vi "Top Level FPGA_noLED.vi"() -> ()   [LabVIEW 2012]
uses:
  <vilib>/Platform/TimedLoop/XDataNode/XDataNode.xnode
  <vilib>/Platform/TimedLoop/XDataNode/nitl_modes.ctl
  <vilib>/Platform/TimedLoop/XDataNode/XDNodeRunTimeDep.lvlib
  <vilib>/Platform/TimedLoop/XDataNode/wakeup.ctl
  <vilib>/Platform/TimedLoop/XDataNode/timing_clust.ctl
  <vilib>/rvi/DataTransferAndStorage/Container/Common/niFpgaContainerMetaDataKey.ctl
  <vilib>/rvi/FIFO/Fifo_Types/niFpgaFifoControlLogicControl.ctl
  <vilib>/rvi/Memory/Memory_Types/niFpgaMemoryInterfaceConfiguration.ctl
  <vilib>/rvi/DataTransferAndStorage/Container/Common/niFpgaContainerInitializationParameters.ctl
  <vilib>/rvi/DataTransferAndStorage/Container/Common/niFpgaTransferTypeControl.ctl
  <vilib>/rvi/DataTransferAndStorage/Container/Common/niFpgaContainerArbitrationOptionsControl.ctl
  <vilib>/rvi/DataTransferAndStorage/Container/Common/niFpgaContainerImplementationControl.ctl
  <vilib>/rvi/DataTransferAndStorage/Container/Common/niFpgaDataTypeControl.ctl
  <vilib>/rvi/DataTransferAndStorage/Container/Common/niFpgaContainerState.ctl
  <vilib>/rvi/DataTransferAndStorage/Container/Common/niFpgaContainerSetEmuInfo.vi
  <vilib>/rvi/eio/common/nirviEmuReportErrorAndStop.vi
  <vilib>/rvi/DataTransferAndStorage/Container/Common/niFpgaContainerGetUniqueNameForEmu.vi
  <vilib>/rvi/LocalResourceManager/LocalResourceManager.xnode
  <vilib>/rvi/DataTransferAndStorage/Container/XNode/niFpgaContainer.xnode
  <vilib>/rvi/Memory/Memory_Emulation/nirvimemoryEmulation.vi
  <vilib>/rvi/FIFO/Fifo_Resource/nirvififoEmulationRead.vi
  <vilib>/rvi/DataTransferAndStorage/Register/Emulation/niFpgaRegisterEmulation.vi
  <vilib>/eio/EIONode/EIONode.xnode
  <vilib>/rvi/eio/common/nirviEmuTemplateMethod_errors.vi
  <vilib>/rvi/FIFO/Fifo_Resource/nirvififoEmulationClear.vi
  <vilib>/rvi/FIFO/Fifo_Resource/nirvififoEmulationWrite.vi
panel:
  out "Timestamp":u64
  in  "Stop FPGA and exit":bool
  out "Exited cleanly?":bool
  out "DMA FIFO Timed Out?":bool
  in  "location":i16(ring) items=["Purdue", "NIKHEF", "Zurich", "???"]
  in  "show_trigger_position_for_debugging":bool
  in  "channel 7 on/off":bool
  in  "channel 6 on/off":bool
  in  "channel 5 on/off":bool
  in  "channel 4 on/off":bool
  in  "channel 3 on/off":bool
  in  "channel 1 on/off":bool
  in  "channel 2 on/off":bool
  in  "channel 0 on/off":bool
  in  "initial value":u64
  in  "circular buffer length":u32=1000
  in  "# of pretrigger":u32=20
  out "IO Module\\Pll Unlocked":bool
  out "IO Module\\ADC Error B":bool
  out "IO Module\\ADC Error A":bool
  out "Init Done":bool
  in  "Simulate":bool
  in  "Trigger 4":i16=4000
  in  "Trigger 5":i16=4000
  in  "Trigger 6":i16=4000
  in  "Trigger 7":i16=4000
  in  "Trigger 2":i16=4000
  in  "Trigger 3":i16=4000
  in  "Trigger 1":i16=4000
  in  "Record Size only data":u32=95
  in  "Trigger 0":i16=4000
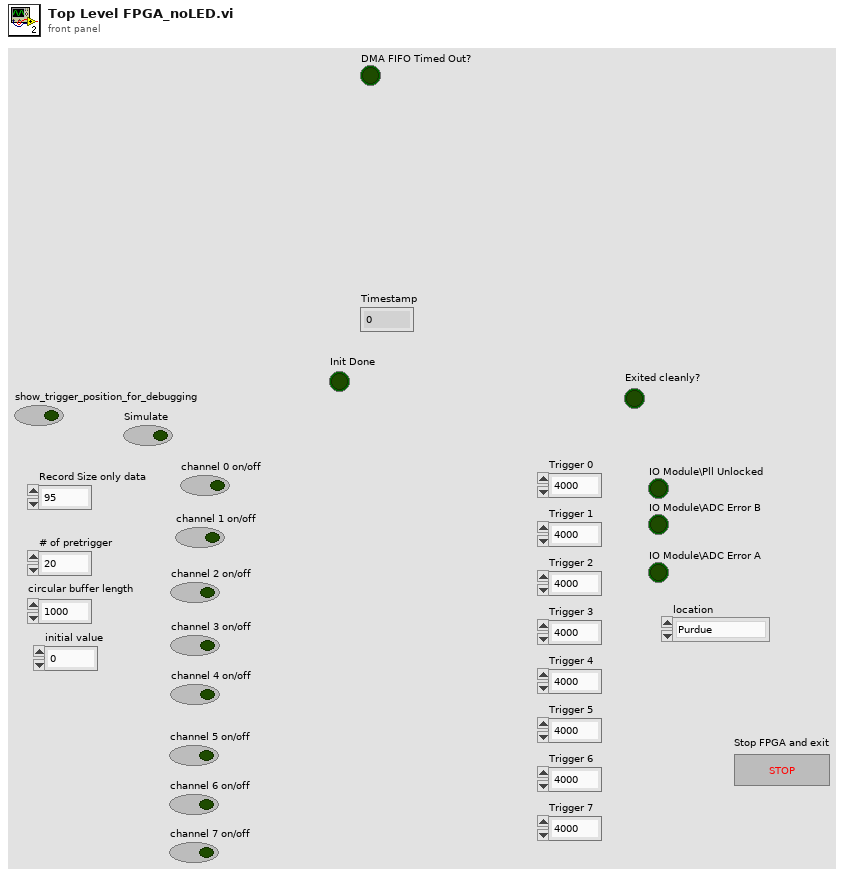
[diagram p1: front panel]
types:
  T1 = typedef "XDNodeRunTimeDep.lvlib/timing_clust.ctl" = cluster{"Expected End [f-1]":u64, "Actual End [f-1]":u64, "Finished Late? [f-1]":bool, "Expected End [i-1]":u64, "Actual End [i-1]":u64, "Finished Late? [i-1]":bool, "Expected Start [i]":u64, "Actual Start [i]":u64, "Expected Start [f]":u64, "Actual Start [f]":u64, "Source Name":string, "Structure Name":string, "Period":i64, "Deadline":i64, "Offset":i64, "Start":i64, "Priority":i32, "Timeout":i32, "Mode":T2, "Wakeup Reason":T3, "Error":errorcluster, "Source Type":string, "Secondary Source Type":string, "Global End Time":u64, "Global Start Time":u64, "Frame Duration":u64, "Iteration Duration":u64, "Assigned CPU":i32, "I/O Scan Engine Mode":u32}
  T2 = typedef "XDNodeRunTimeDep.lvlib/nitl_modes.ctl" = enum32{"No Change", "Process missed periods, maintain original phase", "Discard missed periods, maintain original phase", "Process missed periods, ignore original phase", "Discard missed periods, ignore original phase"}
  T3 = typedef "XDNodeRunTimeDep.lvlib/wakeup.ctl" = enum32{"Normal", "Aborted", "Asynchronous wakeup", "Timing source error", "Timed loop error", "Timeout"}
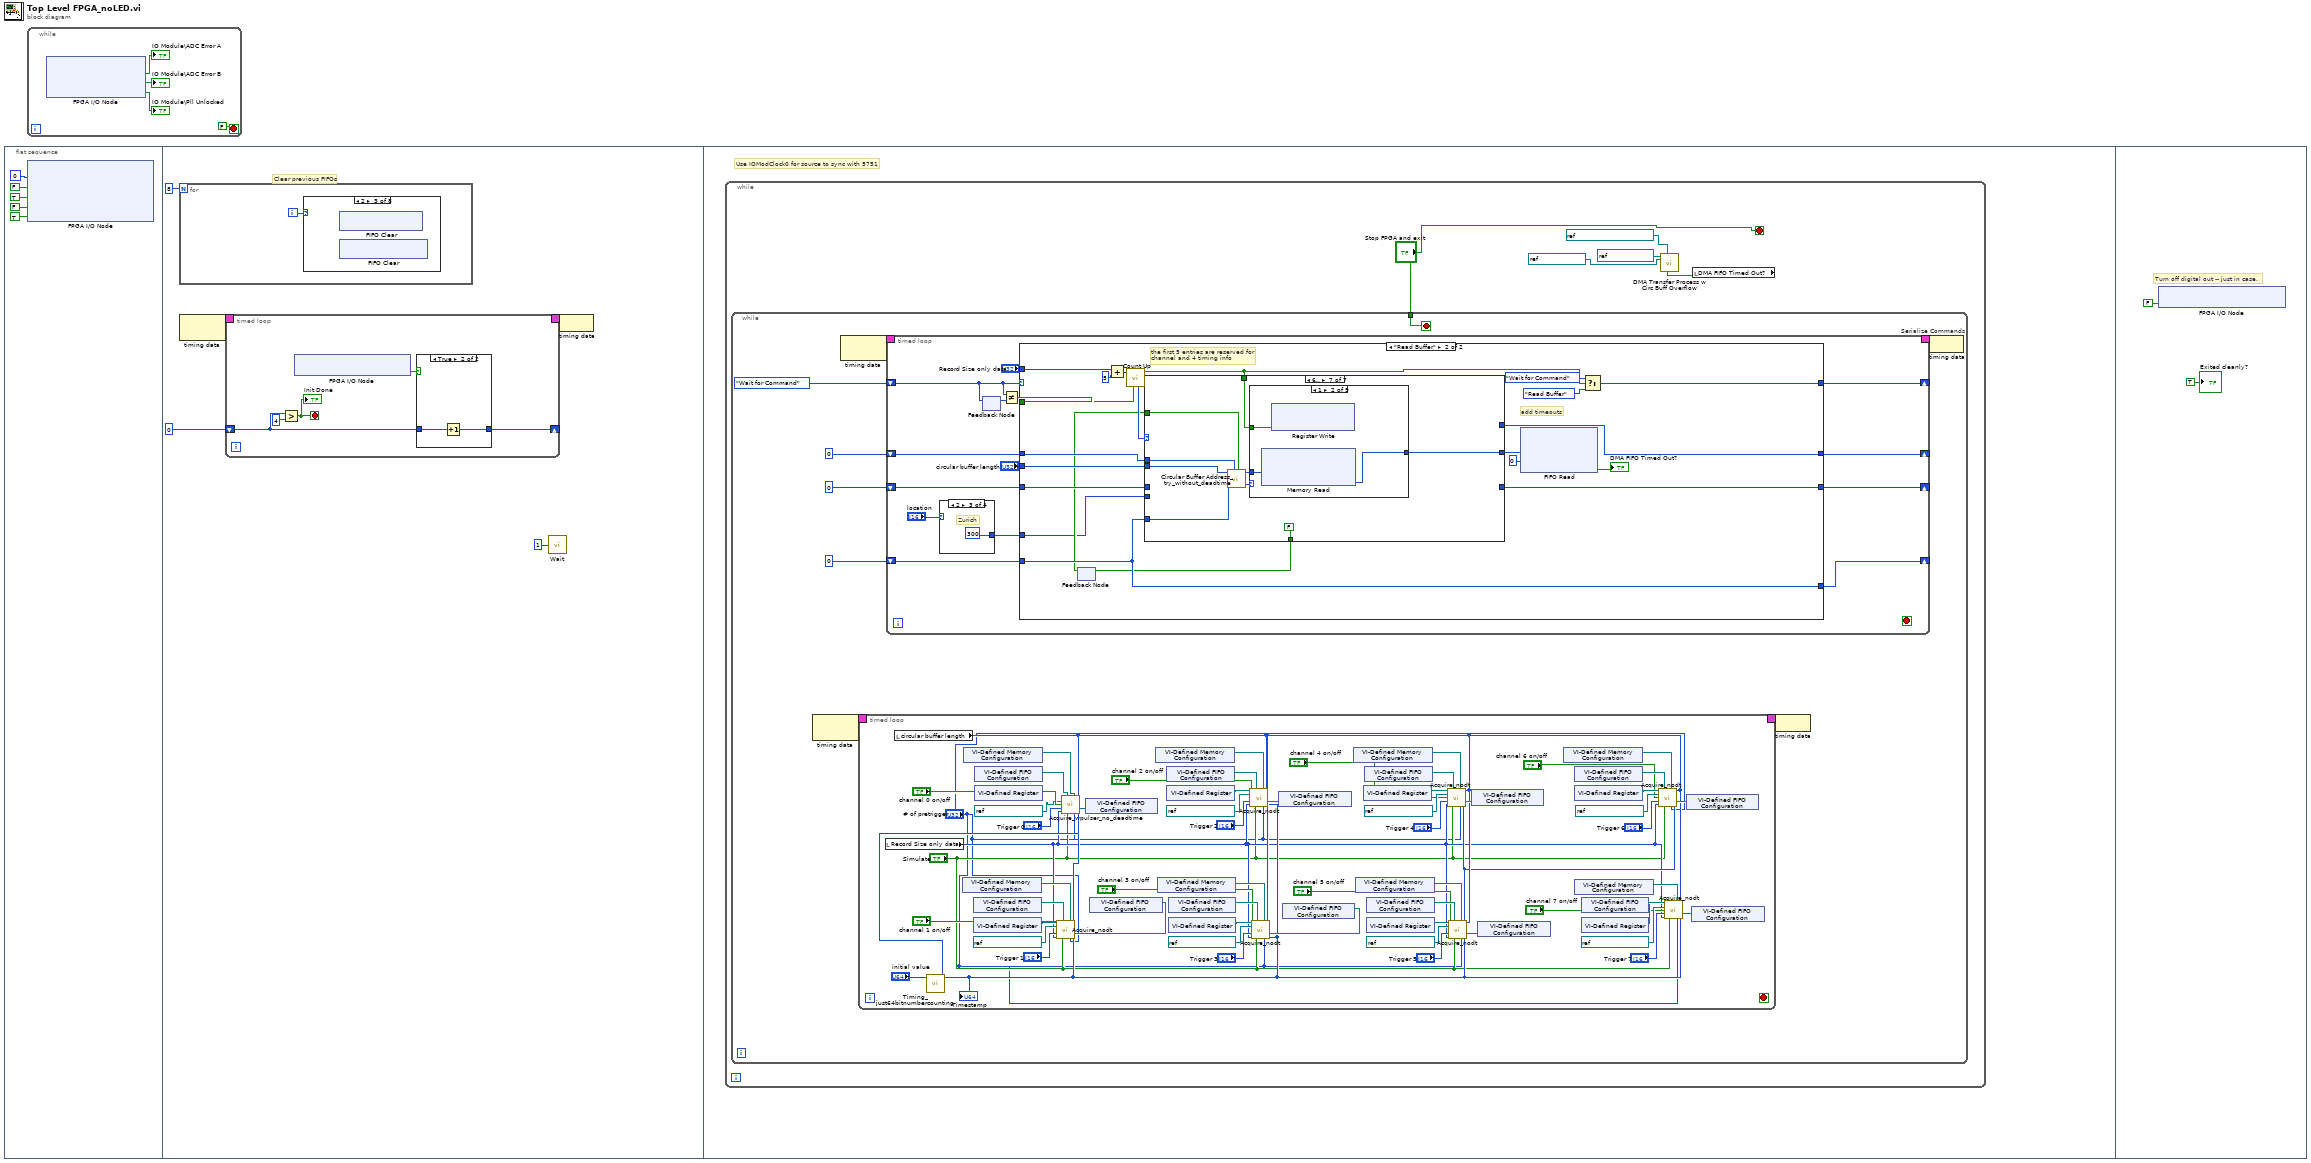
[diagram p0: block diagram]
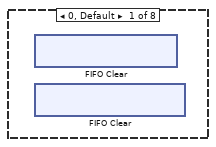
[diagram p2: hidden frame]
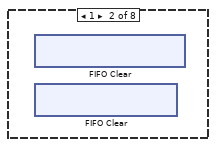
[diagram p3: hidden frame]
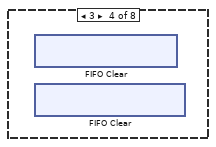
[diagram p4: hidden frame]
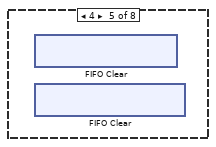
[diagram p5: hidden frame]
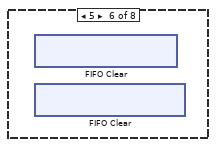
[diagram p6: hidden frame]
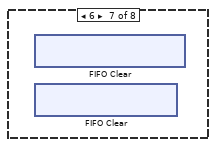
[diagram p7: hidden frame]
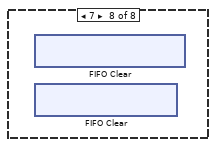
[diagram p8: hidden frame]
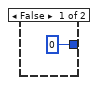
[diagram p9: hidden frame]
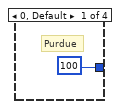
[diagram p10: hidden frame]
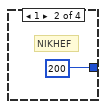
[diagram p11: hidden frame]
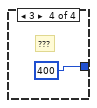
[diagram p12: hidden frame]
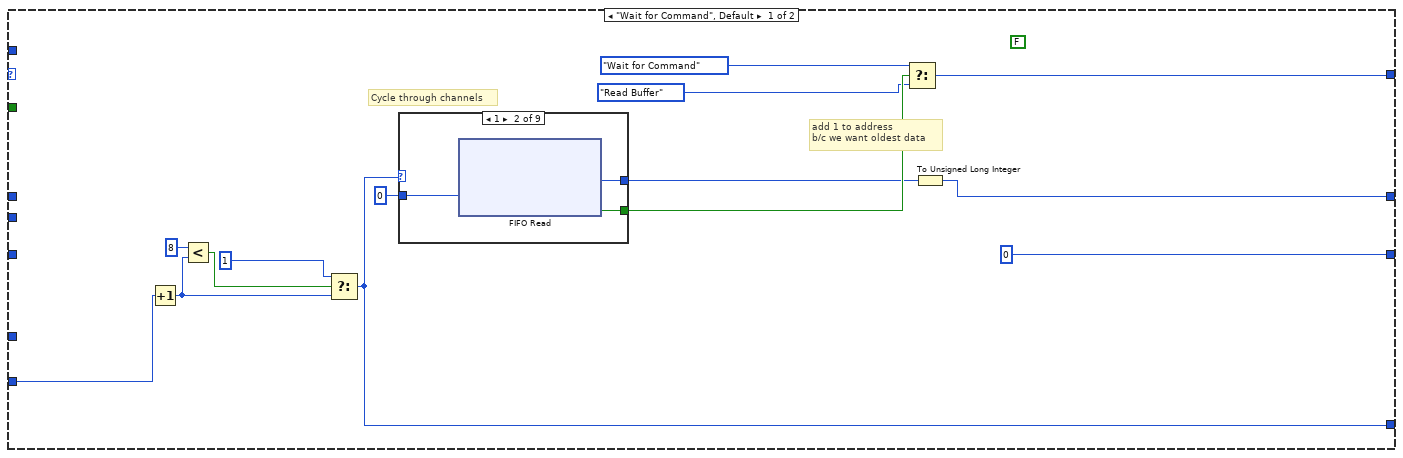
[diagram p13: hidden frame]
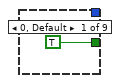
[diagram p14: hidden frame]
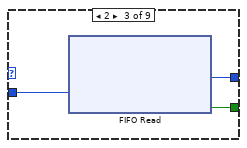
[diagram p15: hidden frame]
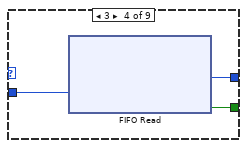
[diagram p16: hidden frame]
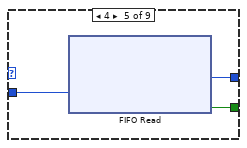
[diagram p17: hidden frame]
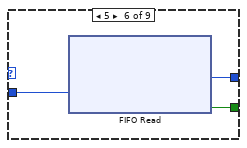
[diagram p18: hidden frame]
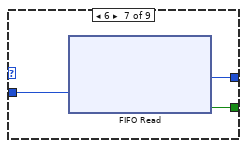
[diagram p19: hidden frame]
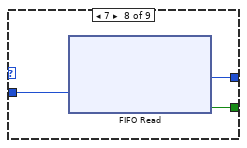
[diagram p20: hidden frame]
diagram:
  n1 = flat-sequence {
    frame #0 {
      n2 = xnode "FPGA I/O Node"("IO Module\\Sample Clock Select"=u8 0 ("IO Module\\Sample Clock Select"), "IO Module\\Force Initialization"=FALSE ("IO Module\\Force Initialization"), "IO Module\\Force Initialization"=TRUE ("IO Module\\Force Initialization"), "IO Module\\Force Initialization"=FALSE ("IO Module\\Force Initialization"), "IO Module\\Digital Output Enable"=TRUE ("IO Module\\Digital Output Enable")) -> ()  [unwired: 5 in, 5 out]
    }
    frame #1 {
      # "Clear previous FIFOs"
      n3 = for {
        N: 8 -> [_]
        i -> [w11]
        n4 = case shown="2" w11 {
          frame 0, Default {
            n5 = xnode ("FIFO Clear")() -> ()  [unwired: 1 in, 1 out]
            n6 = xnode ("FIFO Clear")() -> ()  [unwired: 1 in, 1 out]
          }
          frame 1 {
            n7 = xnode ("FIFO Clear")() -> ()  [unwired: 1 in, 1 out]
            n8 = xnode ("FIFO Clear")() -> ()  [unwired: 1 in, 1 out]
          }
          frame 2 {
            n9 = xnode ("FIFO Clear")() -> ()  [unwired: 1 in, 1 out]
            n10 = xnode ("FIFO Clear")() -> ()  [unwired: 1 in, 1 out]
          }
          frame 3 {
            n11 = xnode ("FIFO Clear")() -> ()  [unwired: 1 in, 1 out]
            n12 = xnode ("FIFO Clear")() -> ()  [unwired: 1 in, 1 out]
          }
          frame 4 {
            n13 = xnode ("FIFO Clear")() -> ()  [unwired: 1 in, 1 out]
            n14 = xnode ("FIFO Clear")() -> ()  [unwired: 1 in, 1 out]
          }
          frame 5 {
            n15 = xnode ("FIFO Clear")() -> ()  [unwired: 1 in, 1 out]
            n16 = xnode ("FIFO Clear")() -> ()  [unwired: 1 in, 1 out]
          }
          frame 6 {
            n17 = xnode ("FIFO Clear")() -> ()  [unwired: 1 in, 1 out]
            n18 = xnode ("FIFO Clear")() -> ()  [unwired: 1 in, 1 out]
          }
          frame 7 {
            n19 = xnode ("FIFO Clear")() -> ()  [unwired: 1 in, 1 out]
            n20 = xnode ("FIFO Clear")() -> ()  [unwired: 1 in, 1 out]
          }
        }
      }
      n21 = node-c288() -> (w10:T1)  [unwired: 1 in]
      n22 = timed-loop {
        shift-right: [w15] -> _
        shift-left: u16 0 -> [w14]
        timing: w10 -> [_]
        timing-out: [_] -> w9
        stop <- w12 stop-if-true
        n23 = Greater?(x=w14, y=u16 4) -> (0:w12:bool)
        "Init Done" <- w12
        n24 = xnode "FPGA I/O Node"() -> ("IO Module\\Initialization Done"=w16:bool)  [unwired: 1 in, 1 out]
        n25 = case shown="True" w16 {
          tunnel: [u16 0 w19] -> w15
          tunnel: w14 -> [_ w18]
          frame False {
          }
          frame True {
            n26 = Increment(x=w18) -> (x+1=w19:u16)
          }
        }
      }
      n27 = call "Wait"("Count(mSec)"=u32 1) -> ()  [unwired: 1 out]
      n28 = node-c288(w9) -> ()
    }
    frame #2 {
      # "Use IOModClock0 for source to sync with 5751"
      n29 = while {
        stop <- "Stop FPGA and exit" stop-if-true
        n30 = while {
          tunnel: "Stop FPGA and exit" -> [w29]
          stop <- w29 stop-if-true
          n31 = node-c288() -> (w35:T1)  [unwired: 1 in]
          n32 = node-c288() -> (w37:T1)  [unwired: 1 in]
          n33 = timed-loop {
            timing: w35 -> [_]
            timing-out: [_] -> w34
            stop <- _ stop-if-true
            n34 = local read "Record Size only data"() -> (w40:u32)
            n35 = local read "circular buffer length"() -> (w42:u32)
            n36 = call "Timing_just64bitnumbercounting.vi"("initial value"="initial value") -> ("x+1"=w41:u64)  [unwired: 10 in]
            "Timestamp" <- w41
            n37 = xnode "VI-Defined Memory Configuration"() -> ("Memory Out"=w97:refnum<k21>)
            n38 = xnode "VI-Defined Memory Configuration"() -> ("Memory Out"=w43:refnum<k21>)
            n39 = xnode "VI-Defined FIFO Configuration"() -> ("FIFO Out"=w96:refnum<k21>)
            n40 = xnode "VI-Defined Register"() -> ("Register Out"=w77:refnum<k21>)
            n41 = xnode "VI-Defined FIFO Configuration"() -> ("FIFO Out"=w44:refnum<k21>)
            n42 = xnode "VI-Defined Register"() -> ()  [unwired: 1 out]
            n43 = xnode "VI-Defined FIFO Configuration"() -> ("FIFO Out"=w48:refnum<k21>)
            n44 = call "Acquire_wpulser_no_deadtime.vi"("Command FIFO"=w44, "Circular Buffer Mem"=w43, "circular buffer length"=w42, "FPGA I/O In"=refnum<k21> "IO Module\\AI A0", "channel\non/off"="channel 0 on/off", "Trigger"="Trigger 0", "Timing FIFO"=w48, "Records to Acquire"=w40, "Simulate"="Simulate", "# of pretrigger"="# of pretrigger", "timing"=w41) -> ()  [unwired: 4 in, 1 out]
            n45 = xnode "VI-Defined FIFO Configuration"() -> ("FIFO Out"=w63:refnum<k21>)
            n46 = call "Acquire_nodt.vi"("Ch Armed Reg"=w77, "Command FIFO"=w96, "Circular Buffer Mem"=w97, "circular buffer length"=w42, "FPGA I/O In"=refnum<k21> "IO Module\\AI A1", "channel on/off"="channel 1 on/off", "Trigger"="Trigger 1", "Timing FIFO"=w63, "Samples to Acquire"=w40, 12:"Simulate", "# of pretrigger"="# of pretrigger", "timing"=w41) -> ()  [unwired: 4 in]
            n47 = xnode "VI-Defined Memory Configuration"() -> ("Memory Out"=w91:refnum<k21>)
            n48 = xnode "VI-Defined Memory Configuration"() -> ("Memory Out"=w94:refnum<k21>)
            n49 = xnode "VI-Defined FIFO Configuration"() -> ("FIFO Out"=w90:refnum<k21>)
            n50 = xnode "VI-Defined Register"() -> ("Register Out"=w73:refnum<k21>)
            n51 = xnode "VI-Defined FIFO Configuration"() -> ("FIFO Out"=w95:refnum<k21>)
            n52 = xnode "VI-Defined Register"() -> ("Register Out"=w75:refnum<k21>)
            n53 = xnode "VI-Defined FIFO Configuration"() -> ("FIFO Out"=w62:refnum<k21>)
            n54 = call "Acquire_nodt.vi"("Ch Armed Reg"=w73, "Command FIFO"=w90, "Circular Buffer Mem"=w91, "circular buffer length"=w42, "FPGA I/O In"=refnum<k21> "IO Module\\AI A2", "channel on/off"="channel 2 on/off", "Trigger"="Trigger 2", "Timing FIFO"=w62, "Samples to Acquire"=w40, 12:"Simulate", "# of pretrigger"="# of pretrigger", "timing"=w41) -> ()  [unwired: 4 in]
            n55 = xnode "VI-Defined FIFO Configuration"() -> ("FIFO Out"=w61:refnum<k21>)
            n56 = call "Acquire_nodt.vi"("Ch Armed Reg"=w75, "Command FIFO"=w95, "Circular Buffer Mem"=w94, "circular buffer length"=w42, "FPGA I/O In"=refnum<k21> "IO Module\\AI A3", "channel on/off"="channel 3 on/off", "Trigger"="Trigger 3", "Timing FIFO"=w61, "Samples to Acquire"=w40, 12:"Simulate", "# of pretrigger"="# of pretrigger", "timing"=w41) -> ()  [unwired: 4 in]
            n57 = xnode "VI-Defined Memory Configuration"() -> ("Memory Out"=w79:refnum<k21>)
            n58 = xnode "VI-Defined Memory Configuration"() -> ("Memory Out"=w82:refnum<k21>)
            n59 = xnode "VI-Defined Register"() -> ("Register Out"=w67:refnum<k21>)
            n60 = xnode "VI-Defined FIFO Configuration"() -> ("FIFO Out"=w78:refnum<k21>)
            n61 = xnode "VI-Defined FIFO Configuration"() -> ("FIFO Out"=w83:refnum<k21>)
            n62 = xnode "VI-Defined Register"() -> ("Register Out"=w71:refnum<k21>)
            n63 = xnode "VI-Defined FIFO Configuration"() -> ("FIFO Out"=w60:refnum<k21>)
            n64 = call "Acquire_nodt.vi"("Ch Armed Reg"=w67, "Command FIFO"=w78, "Circular Buffer Mem"=w79, "circular buffer length"=w42, "FPGA I/O In"=refnum<k21> "IO Module\\AI A4", "channel on/off"="channel 4 on/off", "Trigger"="Trigger 4", "Timing FIFO"=w60, "Samples to Acquire"=w40, 12:"Simulate", "# of pretrigger"="# of pretrigger", "timing"=w41) -> ()  [unwired: 4 in]
            n65 = xnode "VI-Defined FIFO Configuration"() -> ("FIFO Out"=w59:refnum<k21>)
            n66 = call "Acquire_nodt.vi"("Ch Armed Reg"=w71, "Command FIFO"=w83, "Circular Buffer Mem"=w82, "circular buffer length"=w42, "FPGA I/O In"=refnum<k21> "IO Module\\AI A5", "channel on/off"="channel 5 on/off", "Trigger"="Trigger 5", "Timing FIFO"=w59, "Samples to Acquire"=w40, 12:"Simulate", "# of pretrigger"="# of pretrigger", "timing"=w41) -> ()  [unwired: 4 in]
            n67 = xnode "VI-Defined Memory Configuration"() -> ("Memory Out"=w88:refnum<k21>)
            n68 = xnode "VI-Defined Memory Configuration"() -> ("Memory Out"=w85:refnum<k21>)
            n69 = xnode "VI-Defined FIFO Configuration"() -> ("FIFO Out"=w89:refnum<k21>)
            n70 = xnode "VI-Defined Register"() -> ("Register Out"=w69:refnum<k21>)
            n71 = xnode "VI-Defined FIFO Configuration"() -> ("FIFO Out"=w84:refnum<k21>)
            n72 = xnode "VI-Defined Register"() -> ("Register Out"=w65:refnum<k21>)
            n73 = xnode "VI-Defined FIFO Configuration"() -> ("FIFO Out"=w58:refnum<k21>)
            n74 = call "Acquire_nodt.vi"("Ch Armed Reg"=w69, "Command FIFO"=w89, "Circular Buffer Mem"=w88, "circular buffer length"=w42, "FPGA I/O In"=refnum<k21> "IO Module\\AI A6", "channel on/off"="channel 6 on/off", "Trigger"="Trigger 6", "Timing FIFO"=w58, "Samples to Acquire"=w40, 12:"Simulate", "# of pretrigger"="# of pretrigger", "timing"=w41) -> ()  [unwired: 4 in]
            n75 = xnode "VI-Defined FIFO Configuration"() -> ("FIFO Out"=w57:refnum<k21>)
            n76 = call "Acquire_nodt.vi"("Ch Armed Reg"=w65, "Command FIFO"=w84, "Circular Buffer Mem"=w85, "circular buffer length"=w42, "FPGA I/O In"=refnum<k21> "IO Module\\AI A7", "channel on/off"="channel 7 on/off", "Trigger"="Trigger 7", "Timing FIFO"=w57, "Samples to Acquire"=w40, 12:"Simulate", "# of pretrigger"="# of pretrigger", "timing"=w41) -> ()  [unwired: 4 in]
          }
          n77 = timed-loop "Serialize Commands" {
            timing: w37 -> [_]
            timing-out: [_] -> w36
            shift-right: [w879] -> _
            shift-left: enum16{"Wait for Command", "Read Buffer"}."Wait for Command" -> [w877]
            shift-right: [w883] -> _
            shift-left: u32 0 ("Element") -> [w882]
            shift-right: [w881] -> _
            shift-left: u8 0 ("t") -> [w880]
            shift-right: [w874] -> _
            shift-left: u64 0 ("Element") -> [w873]
            stop <- _ stop-if-true
            n78 = case shown="2" "location" {
              tunnel: [i16 100 i16 200 i16 300 i16 400] -> w871
              frame 0, Default {
                # "Purdue"
              }
              frame 1 {
                # "NIKHEF"
              }
              frame 2 {
                # "Zurich"
              }
              frame 3 {
                # "???"
              }
            }
            n79 = feedback-in #1(w877) -> ()
            n80 = feedback #1() -> (w878:enum16{"Wait for Command", "Read Buffer"})  [unwired: 1 in]
            n81 = Not Equal?(x=w877, y=w878) -> (x != y?=w875:bool)
            n82 = case shown="\"Read Buffer\"" w877 {
              tunnel: "Record Size only data" -> [_ w937]
              tunnel: [w891 w947] -> w881
              tunnel: w880 -> [w893 w947]
              tunnel: [w894 w932] -> w883
              tunnel: w882 -> [_ w946]
              tunnel: [w897 w948] -> w879
              tunnel: "circular buffer length" -> [_ w945]
              tunnel: w875 -> [_ w939]
              tunnel: [u64 0 ("Element") w934] -> w874
              tunnel: w873 -> [_ w933]
              tunnel: w871 -> [_ w928]
              frame "Wait for Command", Default {
                (unwired) FALSE
                # "add 1 to address\nb/c we want oldest data"
                # "Cycle through channels"
                n83 = Increment(x=w893) -> (x+1=w892:u8)
                n84 = Less?(x=u8 8, y=w892) -> (x < y?=w901:bool)
                n85 = Select(t=u8 1, s=w901, f=w892) -> (s? t:f=w891:u8)
                n86 = case shown="1" w891 {
                  tunnel: [TRUE ("Timed Out?") w906 w907 w910 w913 w916 w919 w922 w925] -> w898
                  tunnel: 0 ("Timeout") -> [_ w905 w909 w912 w915 w918 w921 w924 w927]
                  tunnel: [_ w904 w908 w911 w914 w917 w920 w923 w926] -> w890
                  frame 0, Default {
                  }
                  frame 1 {
                    n87 = xnode ("FIFO Read")("Timeout"=w905) -> ("Element"=w904:i16, "Timed Out?"=w906:bool)  [unwired: 1 in, 1 out]
                  }
                  frame 2 {
                    n88 = xnode ("FIFO Read")("Timeout"=w909) -> ("Element"=w908:i16, "Timed Out?"=w907:bool)  [unwired: 1 in, 1 out]
                  }
                  frame 3 {
                    n89 = xnode ("FIFO Read")("Timeout"=w912) -> ("Element"=w911:i16, "Timed Out?"=w910:bool)  [unwired: 1 in, 1 out]
                  }
                  frame 4 {
                    n90 = xnode ("FIFO Read")("Timeout"=w915) -> ("Element"=w914:i16, "Timed Out?"=w913:bool)  [unwired: 1 in, 1 out]
                  }
                  frame 5 {
                    n91 = xnode ("FIFO Read")("Timeout"=w918) -> ("Element"=w917:i16, "Timed Out?"=w916:bool)  [unwired: 1 in, 1 out]
                  }
                  frame 6 {
                    n92 = xnode ("FIFO Read")("Timeout"=w921) -> ("Element"=w920:i16, "Timed Out?"=w919:bool)  [unwired: 1 in, 1 out]
                  }
                  frame 7 {
                    n93 = xnode ("FIFO Read")("Timeout"=w924) -> ("Element"=w923:i16, "Timed Out?"=w922:bool)  [unwired: 1 in, 1 out]
                  }
                  frame 8 {
                    n94 = xnode ("FIFO Read")("Timeout"=w927) -> ("Element"=w926:i16, "Timed Out?"=w925:bool)  [unwired: 1 in, 1 out]
                  }
                }
                n95 = Select(t=enum16{"Wait for Command", "Read Buffer"}."Wait for Command", s=w898, f=enum16{"Wait for Command", "Read Buffer"}."Read Buffer") -> (s? t:f=w897:enum16{"Wait for Command", "Read Buffer"})
                n96 = To Unsigned Long Integer(number=w890) -> (unsigned 32bit integer=w894:u32)
              }
              frame "Read Buffer" {
                # "the first 5 entries are reserved for channel and 4 timing info"
                # "add timeouts"
                n97 = feedback #2() -> (w931:bool)  [unwired: 1 in]
                n98 = Add(x=w937, y=u32 5) -> (x+y=w935:u32)
                n99 = call "Count Up.vi"("Reset?"=w939, "goal"=w935) -> ("Count Met"=w941:bool, "count"=w938:u32)  [unwired: 8 in]
                n100 = case shown="6.." w938 {
                  tunnel: w947 -> [_ w955 w962 _ _ _ w1010]
                  tunnel: w946 -> [_ w961 w964 w994 w1000 w1006 w1017]
                  tunnel: w945 -> [_ _ _ _ _ _ w1016]
                  tunnel: w941 -> [_ _ _ _ _ _ w1015]
                  tunnel: [i16 0 ("Data") w958 w968 w992 w998 w1004 w1011] -> w940
                  tunnel: w931 -> [_ _ _ _ _ _ w1013]
                  tunnel: [u64 0 ("Element") _ w967 w995 w1001 w1007 _] -> w934
                  tunnel: w933 -> [_ _ _ w995 w1001 w1007 _]
                  tunnel: [u32 0 ("Element") w961 w964 w994 w1000 w1006 _] -> w932
                  tunnel: [FALSE FALSE FALSE FALSE FALSE TRUE FALSE] -> w930
                  tunnel: w928 -> [_ w953 _ _ _ _ _]
                  frame 0, Default {
                  }
                  frame 1 {
                    w957 = u16 0 items=["Header Information", "Particle Pulse", "Test Pulse"] ("Pulse Type")
                    n101 = Decrement(x=w955) -> (x-1=w956:u8)
                    n102 = To Word Integer(number=w956) -> (16bit integer=w954:i16)
                    n103 = Add(x=w953, y=w954) -> (x+y=w959:i16)
                    n104 = call "bitmanip.vi"("Pulse Type"=w957, "Integer to be written"=w959) -> ("Integer Written"=w958:i16)  [unwired: 2 in]
                  }
                  frame 2 {
                    n105 = case shown="2" w962 {
                      tunnel: [_ w969 w971 w973 w975 w977 w979 w981 w983] -> w963
                      frame Default {
                      }
                      frame 1 {
                        n106 = xnode ("FIFO Read")("Timeout"=0) -> ("Element"=w969:u64)  [unwired: 1 in, 2 out]
                      }
                      frame 2 {
                        n107 = xnode ("FIFO Read")("Timeout"=0) -> ("Element"=w971:u64)  [unwired: 1 in, 2 out]
                      }
                      frame 3 {
                        n108 = xnode ("FIFO Read")("Timeout"=0) -> ("Element"=w973:u64)  [unwired: 1 in, 2 out]
                      }
                      frame 4 {
                        n109 = xnode ("FIFO Read")("Timeout"=0) -> ("Element"=w975:u64)  [unwired: 1 in, 2 out]
                      }
                      frame 5 {
                        n110 = xnode ("FIFO Read")("Timeout"=0) -> ("Element"=w977:u64)  [unwired: 1 in, 2 out]
                      }
                      frame 6 {
                        n111 = xnode ("FIFO Read")("Timeout"=0) -> ("Element"=w979:u64)  [unwired: 1 in, 2 out]
                      }
                      frame 7 {
                        n112 = xnode ("FIFO Read")("Timeout"=0) -> ("Element"=w981:u64)  [unwired: 1 in, 2 out]
                      }
                      frame 8 {
                        n113 = xnode ("FIFO Read")("Timeout"=0) -> ("Element"=w983:u64)  [unwired: 1 in, 2 out]
                      }
                    }
                    n114 = case shown="False" "show_trigger_position_for_debugging" {
                      tunnel: [w985 w989] -> w968
                      tunnel: [w987 w990] -> w967
                      tunnel: w964 -> [_ w991]
                      tunnel: w963 -> [w987 w990]
                      frame False {
                        # "reads out the lsb of the timing information"
                        n115 = Split Number(x=w987) -> (hi(x)=w988:u32)  [unwired: 1 out]
                        n116 = Split Number(x=w988) -> (hi(x)=w986:u16)  [unwired: 1 out]
                        n117 = To Word Integer(number=w986) -> (16bit integer=w985:i16)
                      }
                      frame True {
                        # "plot trigger position instead of the first timing bin"
                        n118 = To Word Integer(number=w991) -> (16bit integer=w989:i16)
                      }
                    }
                  }
                  frame 3 {
                    n119 = Split Number(x=w995) -> (hi(x)=w997:u32)  [unwired: 1 out]
                    n120 = Split Number(x=w997) -> (lo(x)=w996:u16)  [unwired: 1 out]
                    n121 = To Word Integer(number=w996) -> (16bit integer=w992:i16)
                  }
                  frame 4 {
                    n122 = Split Number(x=w1001) -> (lo(x)=w1003:u32)  [unwired: 1 out]
                    n123 = Split Number(x=w1003) -> (hi(x)=w1002:u16)  [unwired: 1 out]
                    n124 = To Word Integer(number=w1002) -> (16bit integer=w998:i16)
                  }
                  frame 5 {
                    n125 = Split Number(x=w1007) -> (lo(x)=w1009:u32)  [unwired: 1 out]
                    n126 = Split Number(x=w1009) -> (lo(x)=w1008:u16)  [unwired: 1 out]
                    n127 = To Word Integer(number=w1008) -> (16bit integer=w1004:i16)
                  }
                  frame 6.. {
                    n128 = call "Circular Buffer Address_try_without_deadtime.vi"("Reset?"=w1013, "Starting Address"=w1017, "circular buffer length"=w1016) -> ("Address"=w1014:u32)  [unwired: 8 in]
                    n129 = case shown="1" w1010 {
                      tunnel: w1014 -> [_ w1021 w1024 w1027 w1030 w1033 w1036 w1039 w1042]
                      tunnel: w1015 -> [_ w1020 w1023 w1026 w1029 w1032 w1035 w1038 w1041]
                      tunnel: [i16 0 w1019 w1022 w1025 w1028 w1031 w1034 w1037 w1040] -> w1011
                      frame Default {
                        # "Error"
                      }
                      frame 1 {
                        n130 = xnode ("Memory Read")("Address"=w1021) -> ("Data"=w1019:i16)  [unwired: 1 in, 1 out]
                        n131 = xnode ("Register Write")("Data"=w1020) -> ()  [unwired: 1 in, 1 out]
                      }
                      frame 2 {
                        n132 = xnode ("Memory Read")("Address"=w1024) -> ("Data"=w1022:i16)  [unwired: 1 in, 1 out]
                        n133 = xnode ("Register Write")("Data"=w1023) -> ()  [unwired: 1 in, 1 out]
                      }
                      frame 3 {
                        n134 = xnode ("Memory Read")("Address"=w1027) -> ("Data"=w1025:i16)  [unwired: 1 in, 1 out]
                        n135 = xnode ("Register Write")("Data"=w1026) -> ()  [unwired: 1 in, 1 out]
                      }
                      frame 4 {
                        n136 = xnode ("Memory Read")("Address"=w1030) -> ("Data"=w1028:i16)  [unwired: 1 in, 1 out]
                        n137 = xnode ("Register Write")("Data"=w1029) -> ()  [unwired: 1 in, 1 out]
                      }
                      frame 5 {
                        n138 = xnode ("Memory Read")("Address"=w1033) -> ("Data"=w1031:i16)  [unwired: 1 in, 1 out]
                        n139 = xnode ("Register Write")("Data"=w1032) -> ()  [unwired: 1 in, 1 out]
                      }
                      frame 6 {
                        n140 = xnode ("Memory Read")("Address"=w1036) -> ("Data"=w1034:i16)  [unwired: 1 in, 1 out]
                        n141 = xnode ("Register Write")("Data"=w1035) -> ()  [unwired: 1 in, 1 out]
                      }
                      frame 7 {
                        n142 = xnode ("Memory Read")("Address"=w1039) -> ("Data"=w1037:i16)  [unwired: 1 in, 1 out]
                        n143 = xnode ("Register Write")("Data"=w1038) -> ()  [unwired: 1 in, 1 out]
                      }
                      frame 8 {
                        n144 = xnode ("Memory Read")("Address"=w1042) -> ("Data"=w1040:i16)  [unwired: 1 in, 1 out]
                        n145 = xnode ("Register Write")("Data"=w1041) -> ()  [unwired: 1 in, 1 out]
                      }
                    }
                  }
                }
                n146 = feedback-in #2(w930) -> ()
                n147 = xnode ("FIFO Read")("Element"=w940, "Timeout"=0) -> ("Timed Out?"=→"DMA FIFO Timed Out?":bool)  [unwired: 1 in, 1 out]
                n148 = Select(t=enum16{"Wait for Command", "Read Buffer"}."Wait for Command", s=w941, f=enum16{"Wait for Command", "Read Buffer"}."Read Buffer") -> (s? t:f=w948:enum16{"Wait for Command", "Read Buffer"})
              }
            }
          }
          n149 = node-c288(w34) -> ()
          n150 = node-c288(w36) -> ()
        }
        n151 = local read "DMA FIFO Timed Out?"() -> (w26:bool)
        n152 = call "DMA Transfer Process w Circ Buff Overflow.vi"("DMA Write Timed Out?"=w26, "Clock Domain"=refnum<k21> "40 MHz Onboard Clock", "Local"=refnum<k21> "To DMA FIFO", "DMA"=refnum<k21> "To Host FIFO") -> ()  [unwired: 8 in]
      }
    }
    frame #3 {
      # "Turn off digital out -- just in case."
      n153 = xnode "FPGA I/O Node"("IO Module\\Digital Output Enable"=FALSE ("IO Module\\Digital Output Enable")) -> ()  [unwired: 1 in, 1 out]
      "Exited cleanly?" <- TRUE ("Exited cleanly?")
    }
  }
  n154 = while {
    stop <- FALSE stop-if-true
    n155 = xnode "FPGA I/O Node"() -> ("IO Module\\ADC Error A"=→"IO Module\\ADC Error A":bool, "IO Module\\ADC Error B"=→"IO Module\\ADC Error B":bool, "IO Module\\Pll Unlocked"=→"IO Module\\Pll Unlocked":bool)  [unwired: 3 in, 3 out]
  }
